vi "Joystick Scaler.vi"(9 "Scaler":dbl, 11 "Joystick Value":dbl) -> (3 "Final Joystick Value":dbl)   [LabVIEW 2019, in "8085 VI Library.lvlib"]
uses:
  8085 VI Library.lvlib
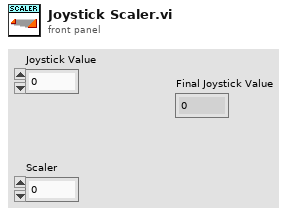
[diagram p1: front panel]
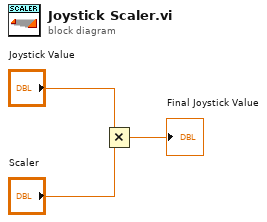
[diagram p0: block diagram]
diagram:
  n1 = Multiply(x="Joystick Value", y="Scaler") -> (x*y=→"Final Joystick Value":dbl)
